vi "Gen Event.vi"(10 "Event Config":T1, 11 "register bus":T2={"Speed"="", "Crank Angle"="", "Cycle Angle"="", "Crank Count"="", "Cycle Count"="", "1.25 MHz Counter"="", "Crank Rollover"="Crank Rollover", "Cycle Rollover"="Cycle Rollover", "shared settings"={"start"=0.0, "stuck limit"=0.0}} {"shared settings"."start" format="%#.15g"}) -> (3 "Event":bool)   [LabVIEW 2013]
uses:
  IP Source/APU/Register Bus.ctl
  IP Source/APU/Shared Settings.ctl
  Event Gen Config.ctl
  <instrlib>/_niInstr/Basic Elements/v1/FPGA/Private/Count Up U32.vi
  <vilib>/rvi/DataTransferAndStorage/Container/Common/niFpgaContainerExecOnDevCompGetState.vi
  <vilib>/rvi/DataTransferAndStorage/Register/Emulation/niFpgaRegisterEmulationFpgaImpl.vi
  <instcachedir>/0/niFpgaRegisterEmulationFpgaImpl_DCF4BC0110594B98B44A971D60CEEC4D.lvgen/niFpgaRegisterEmulationFpgaImpl_DCF4BC0110594B98B44A971D60CEEC4D_006.vi
  <vilib>/rvi/DataTransferAndStorage/Container/Common/niFpgaContainerGetUniqueNameForEmu.vi
  <vilib>/rvi/DataTransferAndStorage/Container/XNode/niFpgaContainer.xnode
  <vilib>/rvi/DataTransferAndStorage/Register/Emulation/niFpgaRegisterEmulationRefIn.vi
  <instrlib>/_niInstr/Basic Elements/v1/FPGA/niInstr Basic Elements v1 FPGA.lvlib
  IP Source/Engine Simulation Toolkit.lvlib
  IP Source/APU/APU.lvlib
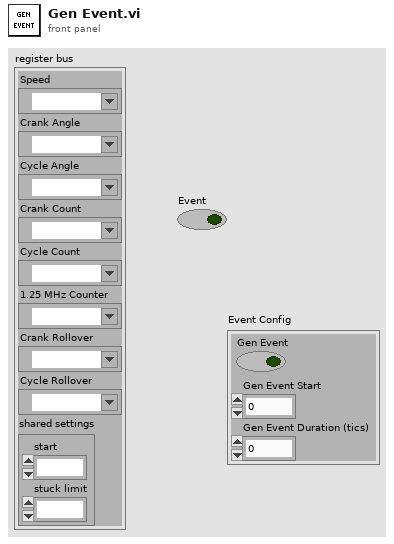
[diagram p1: front panel]
types:
  T1 = typedef "Event Gen Config.ctl" = cluster{"Gen Event":bool, "Gen Event Start":u16, "Gen Event Duration (tics)":u32}
  T2 = typedef "Engine Simulation Toolkit.lvlib/APU.lvlib/Register Bus.ctl" = cluster{"Speed":refnum<k21>, "Crank Angle":refnum<k21>, "Cycle Angle":refnum<k21>, "Crank Count":refnum<k21>, "Cycle Count":refnum<k21>, "1.25 MHz Counter":refnum<k21>, "Crank Rollover":refnum<k21>, "Cycle Rollover":refnum<k21>, "shared settings":T3}
  T3 = typedef "Engine Simulation Toolkit.lvlib/APU.lvlib/Shared Settings.ctl" = cluster{"start":fxp<+,17,17>, "stuck limit":fxp<+,18,18>}
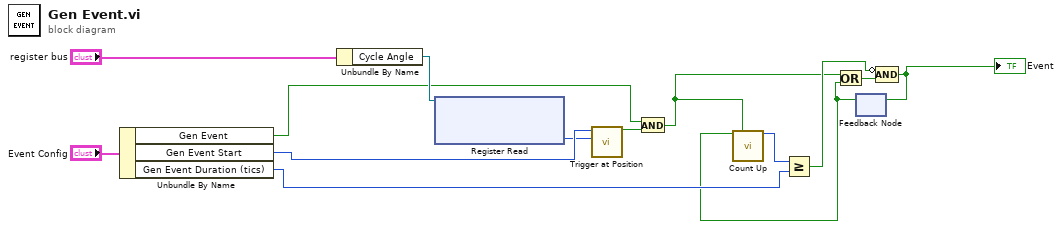
[diagram p0: block diagram]
diagram:
  n1 = Unbundle By Name("Event Config") -> ("Gen Event"=w1:bool, "Gen Event Start"=w12:u16, "Gen Event Duration (tics)"=w11:u32)
  n2 = Unbundle By Name("register bus") -> ("Cycle Angle"=w9:refnum<k21>)
  n3 = xnode "Register Read"("Register In"=w9) -> ("Data"=w7:u16)  [unwired: 1 out]
  n4 = call "Trigger at Position.vi"("position"=w7, "trigger position"=w12) -> ("trigger"=w5:bool)  [unwired: 9 in]
  n5 = And(x=w1, y=w5) -> (x .and. y?=w2:bool)
  n6 = feedback #1() -> (w3:bool)  [unwired: 1 in]
  n7 = call-poly <instrlib>:"Count Up.vi"("increment"=w3, "reset"=w2) -> ("count out"=w8:u32)  [unwired: 13 in]
  n8 = Greater Or Equal?(x=w8, y=w11) -> (x >= y?=w4:bool)
  n9 = Or(x=w2, y=w3) -> (x .or. y?=w6:bool)
  n10 = Compound Arithmetic op=AND(invert w4, w6) -> (w10:bool)
  "Event" <- w10
  n11 = feedback-in #1(w10) -> ()
